vi "Duzy wykres FGV.vi"(7 "Akcja":T1, 8 "error in (no error)":errorcluster, 10 "Okno1 in":bool) -> (0 "error out":errorcluster, 2 "Okno1 out":bool)   [LabVIEW 2014]
doc: "Use this template to build a VI to use as a subVI."
uses:
  Kontrolki/FVGs/FVG akcje podstawowa.ctl
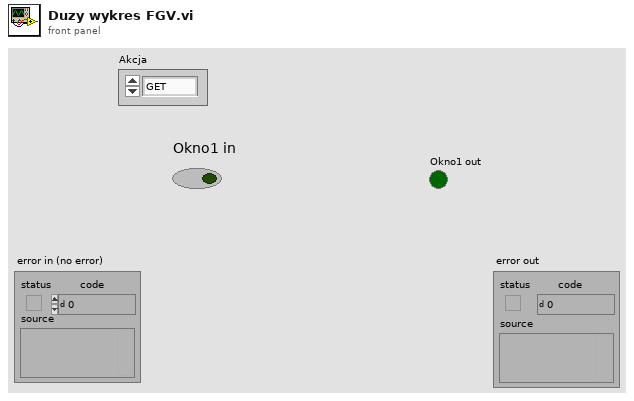
[diagram p1: front panel]
types:
  T1 = typedef "FVG akcje podstawowa.ctl" = enum16{"GET", "SET"}
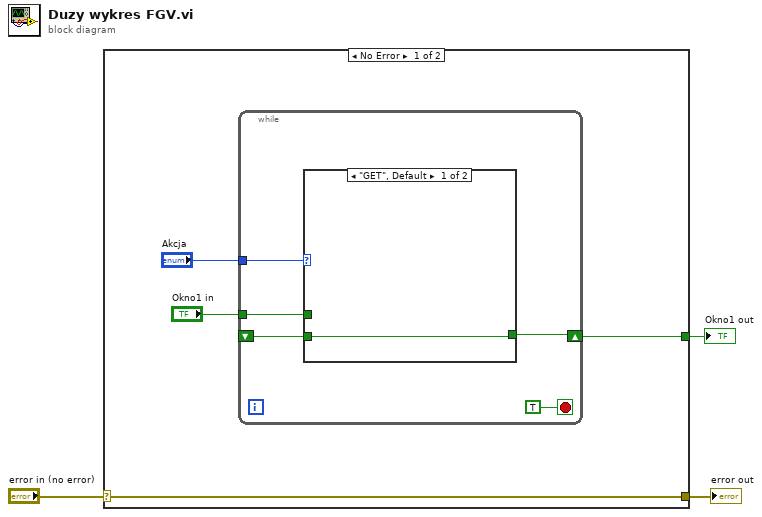
[diagram p0: block diagram]
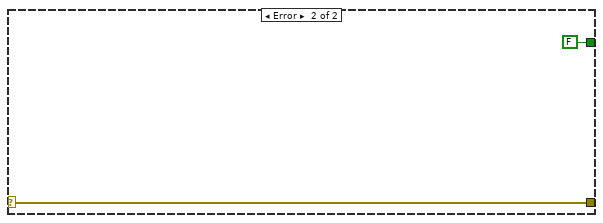
[diagram p3: hidden frame]
diagram:
  n1 = case shown="No Error" "error in (no error)" {
    selector: "error in (no error)" -> [w5 w16]
    tunnel: [w5 w16] -> w2
    tunnel: [w4 FALSE ("Okno in")] -> w1
    frame No Error {
      n2 = while {
        tunnel: "Akcja" -> [w12]
        tunnel: "Okno1 in" -> [w11]
        shift-right: [w10] -> w4
        shift-left: _ -> [w9]
        stop <- TRUE stop-if-true
        n3 = case shown="\"GET\", Default" w12 {
          tunnel: w11 -> [_ w14]
          tunnel: [w13 w14] -> w10
          tunnel: w9 -> [w13 _]
          frame "GET", Default {
          }
          frame "SET" {
          }
        }
      }
    }
    frame Error {
    }
  }
  "error out" <- w2
  "Okno1 out" <- w1
